vi "SendUIMessage.vi"(8 "error in (no error)":errorcluster, 9 "UIMsg":T1, 11 "SendMessage in":refnum<class "SendMessage.lvclass">) -> (0 "error out":errorcluster, 3 "SendMessage out":refnum<class "SendMessage.lvclass">)   [LabVIEW 2019, in "SendMessage.lvclass"]
doc: "Post UI Meessage to Main UI Que.\nShould not post if Error In = True"
uses:
  SendMessage.lvclass
  Support/MessageAPI/UIMessage.ctl
  SendMessage.lvclass/SendMessage.ctl
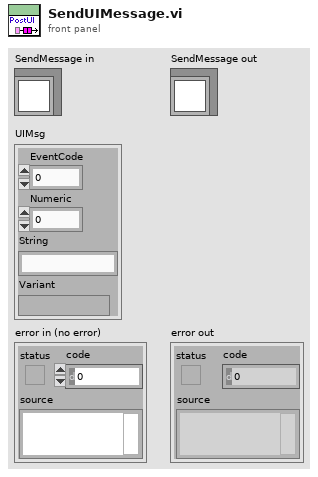
[diagram p1: front panel]
types:
  T1 = typedef "UIMessage.ctl" = cluster{"EventCode":i32, "Numeric":dbl, "String":string, "Variant":variant}
  T2 = typedef "MessageQue.lvlib/MessageQue.ctl" = refnum<queue>
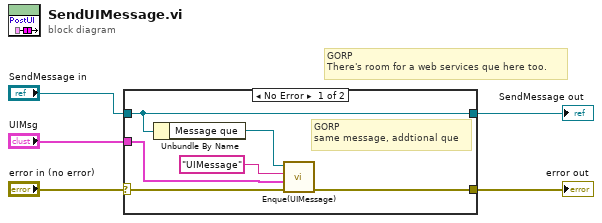
[diagram p0: block diagram]
diagram:
  # "GORP\nThere's room for a web services que here too."
  n1 = case shown="No Error" "error in (no error)" {
    selector: "error in (no error)" -> [w7 w13]
    tunnel: [w6 w13] -> w4
    tunnel: [w11 w12] -> w2
    tunnel: "SendMessage in" -> [w11 w12]
    tunnel: "UIMsg" -> [w8 _]
    frame No Error {
      # "GORP\nsame message, addtional que"
      n2 = Unbundle By Name(w11) -> ("Message que"=w10:T2)
      n3 = call "Enque(UIMessage).vi"("error in"=w7, "UIMsg"=w8, "Message Command"="UIMessage", "Message que"=w10) -> ("error out"=w6:errorcluster)  [unwired: 6 in, 1 out]
    }
    frame Error {
    }
  }
  "error out" <- w4
  "SendMessage out" <- w2
